vi "solar_cfg Write (Ref).vi"(0 "Config Refnum":refnum<data-value>, 1 "Section":string, 2 "Comments (Key,Comment)":cluster{"Key":string, "Comment":string}[](array[cluster]), 5 "Key_Prefix (\"\")":string, 7 "Ctrl Refnum":refnum<vi>, 11 "error in (no error)":errorcluster, 12 "ArrayDelimiters (1D,2D)":string[](array[string])) -> (4 "dup Config Refnum":refnum<data-value>, 10 "Found?":bool, 15 "error out":errorcluster)   [LabVIEW 2018]
doc: "Write the values associated with a control reference to a specified section in the configuration file. If the Key is empty the control reference label is used instead. Set a Comment (#...) to add a description after the key's value. Clusters use the element lables are their key names. Set Enum as Strings to True to use the string item of an enum.\n\nSupported Data Types: \nI8..EXT, Enum, Boolean, String, Path, VISA Reference, Timestamp\n1D & 2D Arrays and Clusters of the data types above.\n\n[Section]\nKey = \"Value\" #Comment"
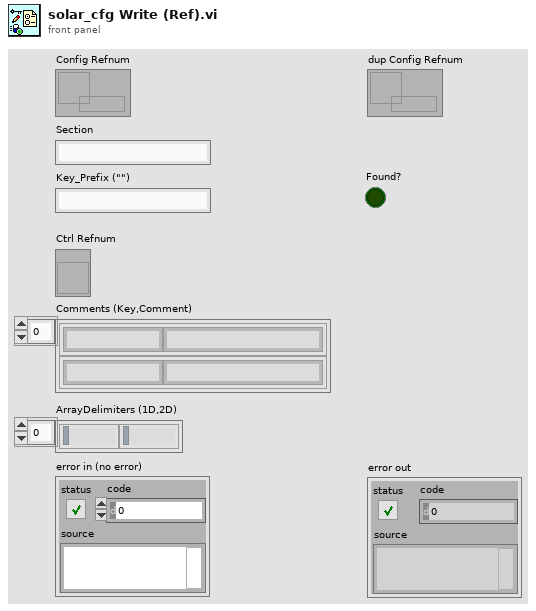
[diagram p1: front panel]
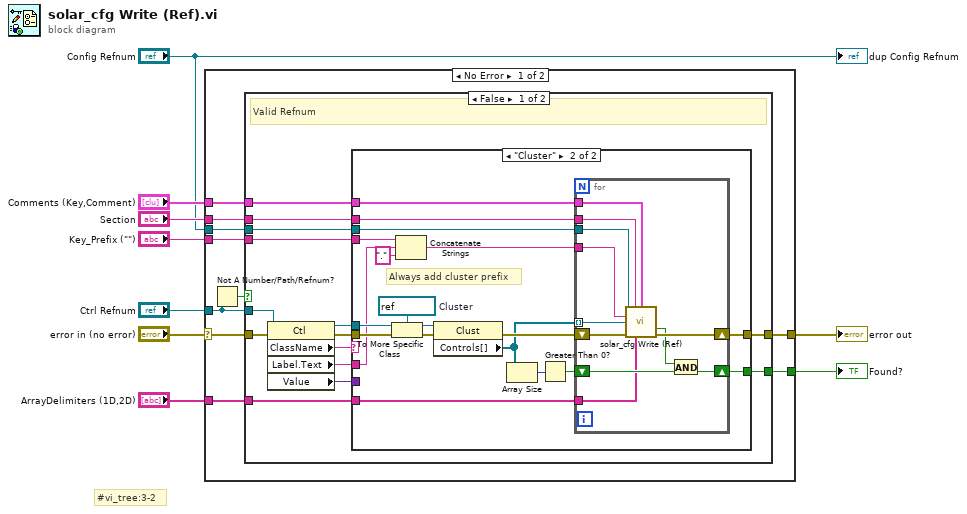
[diagram p0: block diagram]
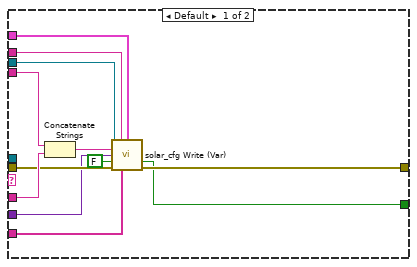
[diagram p2: hidden frame]
diagram:
  # "#vi_tree:3-2"
  n1 = case shown="No Error" "error in (no error)" {
    selector: "error in (no error)" -> [w14 w77]
    tunnel: [w12 w77] -> w8
    tunnel: "Section" -> [w18 _]
    tunnel: "Ctrl Refnum" -> [w15 _]
    tunnel: "Key_Prefix (\"\")" -> [w17 _]
    tunnel: "Comments (Key,Comment)" -> [w19 _]
    tunnel: "ArrayDelimiters (1D,2D)" -> [w13 _]
    tunnel: "Config Refnum" -> [w16 _]
    tunnel: [w11 _] -> w1
    frame No Error {
      n2 = Not A Number/Path/Refnum?(number/path/refnum=w15) -> (NaN/Path/Refnum?=w10:bool)
      n3 = case "Invalid Refnum?" shown="False" w10 {
        tunnel: w14 -> [w26 w76]
        tunnel: w15 -> [w24 _]
        tunnel: [w27 w76] -> w12
        tunnel: w17 -> [w28 _]
        tunnel: w16 -> [w33 _]
        tunnel: [w32 _] -> w11
        tunnel: w18 -> [w31 _]
        tunnel: w13 -> [w30 _]
        tunnel: w19 -> [w29 _]
        frame False {
          # "Valid Refnum"
          n4 = property class="Ctl"(reference=w24, error in=w26) -> (reference out=w20:refnum<vi>, error out=w25:errorcluster, "ClassName"=w23:string, "Label.Text"=w22:string, "Value"=w21:variant)
          n5 = case shown="\"Cluster\"" w23 {
            tunnel: w33 -> [w39 w57]
            tunnel: [w36 w47] -> w32
            tunnel: w31 -> [w38 w56]
            tunnel: w30 -> [w35 w51]
            tunnel: w29 -> [w37 w55]
            tunnel: w28 -> [w44 w58]
            tunnel: w25 -> [w43 w61]
            tunnel: [w40 w46] -> w27
            tunnel: w22 -> [w45 w53]
            tunnel: w21 -> [w42 _]
            tunnel: w20 -> [_ w60]
            frame Default {
              n6 = Concatenate Strings(w44, w45) -> (w41:string)
              n7 = call "solar_cfg Write (Var).vi"("Config Refnum"=w39, "Section"=w38, "Comments (Key,Comment)"=w37, "Key (\"\")"=w41, "Variant"=w42, "Include Variant Name? (F)"=FALSE ("Include Cluster Name? (F)"), "error in (no error)"=w43, "ArrayDelimiters (1D,2D)"=w35) -> ("Found?"=w36:bool, "error out"=w40:errorcluster)  [unwired: 5 in, 1 out]
            }
            frame "Cluster" {
              w63 = refnum<vi> refnum  # Cluster
              # "Always add cluster prefix"
              n8 = To More Specific Class(target class=w63, reference=w60, error in=w61) -> (specific class reference=w64:refnum<vi>, error out=w62:errorcluster)
              n9 = Concatenate Strings(w58, w53, "." ("string")) -> (w54:string)
              n10 = property class="Clust"(reference=w64, error in=w62) -> (error out=w59:errorcluster, "Controls[]"=w50:refnum<vi>[])  [unwired: 1 out]
              n11 = Array Size(array=w50) -> (size(s)=w49:i32)
              n12 = Greater Than 0?(x=w49) -> (x > 0?=w48:bool)
              n13 = for {
                tunnel: w57 -> [w71]
                tunnel: w56 -> [w69]
                tunnel: w55 -> [w68]
                tunnel: w54 -> [w70]
                tunnel: w50 -> [w72] mode=indexing
                shift-right: [w66] -> w46
                shift-left: w59 -> [w73]
                tunnel: w51 -> [w67]
                shift-right: [w74] -> w47
                shift-left: w48 -> [w75]
                n14 = call "solar_cfg Write (Ref).vi"("Config Refnum"=w71, "Section"=w69, "Comments (Key,Comment)"=w68, "Key_Prefix (\"\")"=w70, "Ctrl Refnum"=w72, "error in (no error)"=w73, "ArrayDelimiters (1D,2D)"=w67) -> ("Found?"=w65:bool, "error out"=w66:errorcluster)  [unwired: 6 in, 1 out]
                n15 = And(x=w65, y=w75) -> (x .and. y?=w74:bool)
              }
            }
          }
        }
        frame True {
          # "Invalid Refnum"
        }
      }
    }
    frame Error {
    }
  }
  "error out" <- w8
  "Found?" <- w1
  "dup Config Refnum" <- "Config Refnum"
